vi "prompt.vi"(0 "Enable":bool=TRUE, 5 "error in (no error)":errorcluster) -> (12 "Measurement":enum16{"TEQ", "POL", "QCV"}(ring)=enum."POL", 13 "Run comment":string, 14 "Q curve comment":string, 15 "Q curve file":string, 16 "TE Comment":string, 17 "TE peak file":string, 18 "OK":bool, 19 "error out":errorcluster)   [LabVIEW 2018]
doc: "Displays a standard dialog box that prompts users to enter information, such as a user name and password.\n--------------------\n\nThis Express VI is configured as follows:\n\nMessage to Display to the User:Enter relevant file for TE curve\nThe inputs are: \nText Entry Box: TE peak file\nText Entry Box: TE Comment\nText Entry Box: Q curve file\nText Entry Box: Q curve comment\nText Entry Box: Run comment\nText Entry Box: QCV, TEQ or POL"
uses:
  Global 2.vi
panel:
  in  "Measurement":enum16{"TEQ", "POL", "QCV"}(ring)=enum."POL"
  in  "Run comment":string
  in  "Q curve comment":string
  in  "Q curve file":string
  in  "TE Comment":string
  in  "TE peak file":string
  out "String":string="Enter relevant file for TE curve"
  in  "Cancel":bool
  in  "OK2":bool
  in  "OK1":bool
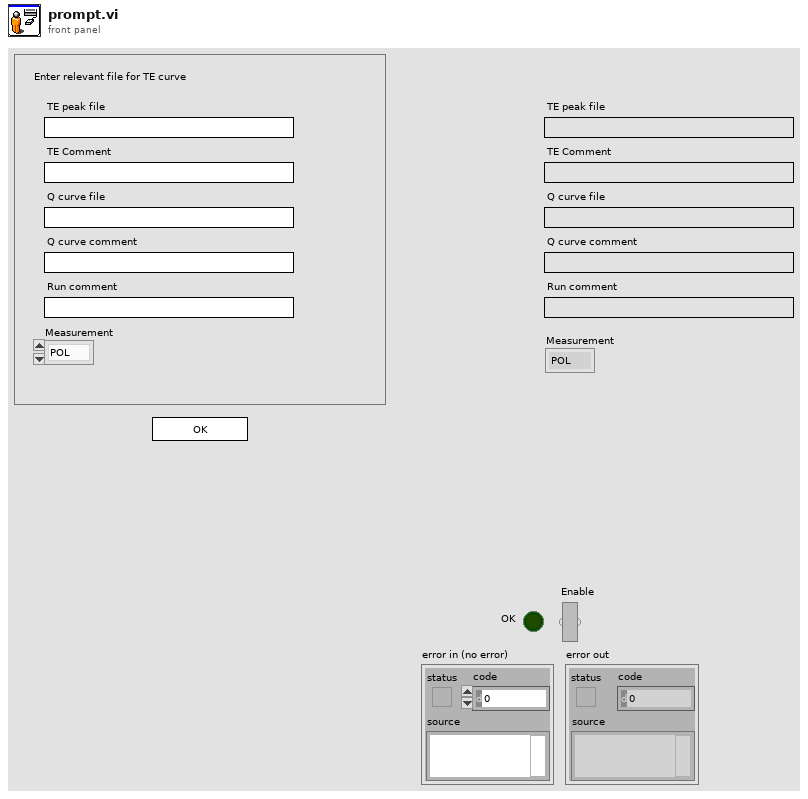
[diagram p1: front panel]
types:
  T1 = cluster{"Input Name":string, "Input Data Type":i32}[]
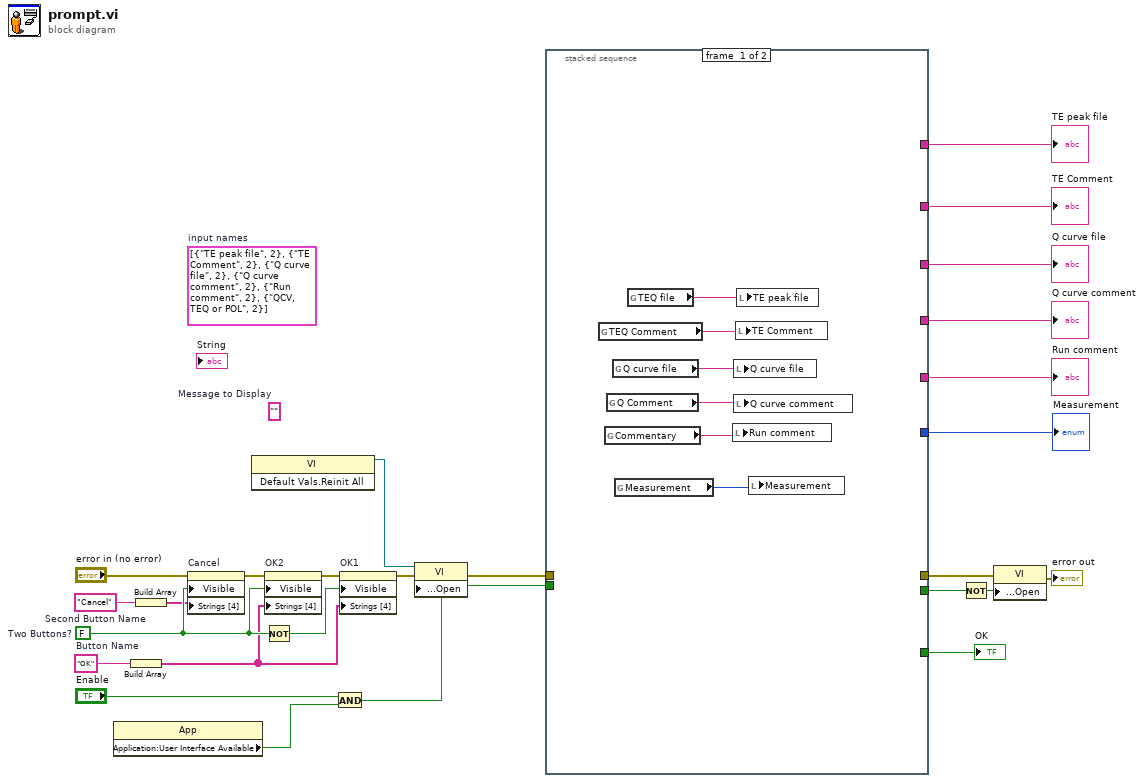
[diagram p0: block diagram]
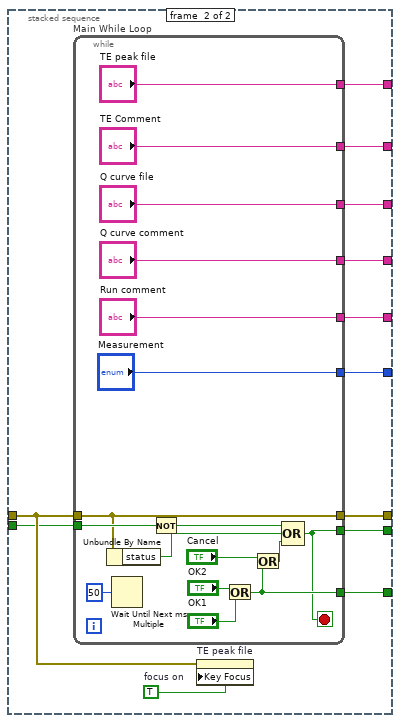
[diagram p2: hidden frame]
diagram:
  (unwired) T1 [{"Input Name"="TE peak file", "Input Data Type"=2}, {"Input Name"="TE Comment", "Input Data Type"=2}, {"Input Name"="Q curve file", "Input Data Type"=2}, {"Input Name"="Q curve comment", "Input Data Type"=2}, {"Input Name"="Run comment", "Input Data Type"=2}, {"Input Name"="QCV, TEQ or POL", "Input Data Type"=2}]  # input names
  w18 = "Cancel"  # Second Button Name
  w16 = "OK"  # Button Name
  (unwired) ""  # Message to Display
  w26 = FALSE  # Two Buttons?
  n1 = property class="App"() -> ("Application:User Interface Available"=w8:bool)  [unwired: 2 in, 2 out]
  n2 = Build Array(w16) -> (w17:string[])
  n3 = Build Array(w18) -> (w19:string[])
  n4 = property on="Cancel" class="Bool"(error in="error in (no error)", "Visible"=w26, "Strings [4]"=w19) -> (error out=w23:errorcluster)  [unwired: 1 in, 1 out]
  n5 = invoke class="VI" method="Default Vals.Reinit All"() -> (reference out=w7:refnum<vi>)  [unwired: 3 in, 2 out]
  n6 = Not(x=w26) -> (.not. x?=w24:bool)
  n7 = property on="OK2" class="Bool"(error in=w23, "Visible"=w26, "Strings [4]"=w17) -> (error out=w22:errorcluster)  [unwired: 1 in, 1 out]
  n8 = And(x="Enable", y=w8) -> (x .and. y?=w9:bool)
  n9 = property on="OK1" class="Bool"(error in=w22, "Visible"=w24, "Strings [4]"=w17) -> (error out=w15:errorcluster)  [unwired: 1 in, 1 out]
  n10 = property class="VI"(reference=w7, error in=w15, "Front Panel Window:Open"=w9) -> (error out=w14:errorcluster)  [unwired: 1 out]
  n11 = stacked-sequence {
    tunnel: [_ w44] -> w25
    tunnel: [_ w43] -> w20
    tunnel: w14 -> [_ w42]
    tunnel: [_ w41] -> w12
    tunnel: w9 -> [_ w40]
    tunnel: [_ w38] -> w6
    tunnel: [_ w37] -> w5
    tunnel: [_ w36] -> w4
    tunnel: [_ w35] -> w3
    tunnel: [_ w34] -> w2
    tunnel: [_ w33] -> w1
    frame #0 {
      n12 = global read "Global 2.vi" "TEQ Comment"() -> (w31:string)
      n13 = global read "Global 2.vi" "Commentary"() -> (w28:string)
      n14 = global read "Global 2.vi" "Q Comment"() -> (w29:string)
      n15 = global read "Global 2.vi" "Q curve file"() -> (w30:string)
      n16 = global read "Global 2.vi" "Measurement"() -> (w27:enum16{"TEQ", "POL", "QCV"})
      n17 = global read "Global 2.vi" "TEQ file"() -> (w32:string)
      n18 = local write "Run comment"(w28) -> ()
      n19 = local write "Q curve file"(w30) -> ()
      n20 = local write "Q curve comment"(w29) -> ()
      n21 = local write "TE Comment"(w31) -> ()
      n22 = local write "TE peak file"(w32) -> ()
      n23 = local write "Measurement"(w27) -> ()
    }
    frame #1 {
      w39 = TRUE  # focus on
      n24 = while "Main While Loop" {
        tunnel: [w58] -> w44
        tunnel: w40 -> [w56]
        tunnel: [w54] -> w43
        tunnel: w42 -> [w53]
        tunnel: [w53] -> w41
        tunnel: ["TE peak file"] -> w38
        tunnel: ["TE Comment"] -> w37
        tunnel: ["Q curve file"] -> w36
        tunnel: ["Q curve comment"] -> w35
        tunnel: ["Run comment"] -> w34
        tunnel: ["Measurement"] -> w33
        stop <- w54 stop-if-true
        n25 = Unbundle By Name(w53) -> ("status"=w51:bool)
        n26 = Wait Until Next ms Multiple(millisecond multiple=u32 50) -> ()  [unwired: 1 out]
        n27 = Not(x=w56) -> (.not. x?=w55:bool)
        n28 = Or(x="OK2", y="OK1") -> (x .or. y?=w58:bool)
        n29 = Or(x="Cancel", y=w58) -> (x .or. y?=w52:bool)
        n30 = Compound Arithmetic op=OR(w55, w51, w52) -> (w54:bool)
      }
      n31 = property on="TE peak file" class="Str"(error in=w42, "Key Focus"=w39) -> ()  [unwired: 1 in, 2 out]
    }
  }
  "OK" <- w25
  "TE peak file" <- w6
  "TE Comment" <- w5
  "Q curve file" <- w4
  "Q curve comment" <- w3
  "Run comment" <- w2
  "Measurement" <- w1
  n32 = Not(x=w20) -> (.not. x?=w21:bool)
  n33 = property class="VI"(error in=w12, "Front Panel Window:Open"=w21) -> (error out=→"error out":errorcluster)  [unwired: 1 in, 1 out]
